vi "Error Converter (ErrCode or Status).vi"(8 "error in (no error)":errorcluster, 11 "error code":i32) -> (0 "error out":errorcluster)   [LabVIEW 2017, in "opcua.lvlib"]
uses:
  opcua.lvlib
panel:
  in  "string":string="This error is returned by the shared library function."
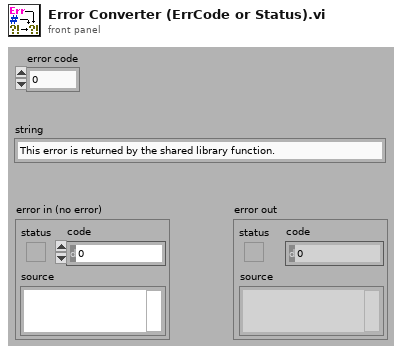
[diagram p1: front panel]
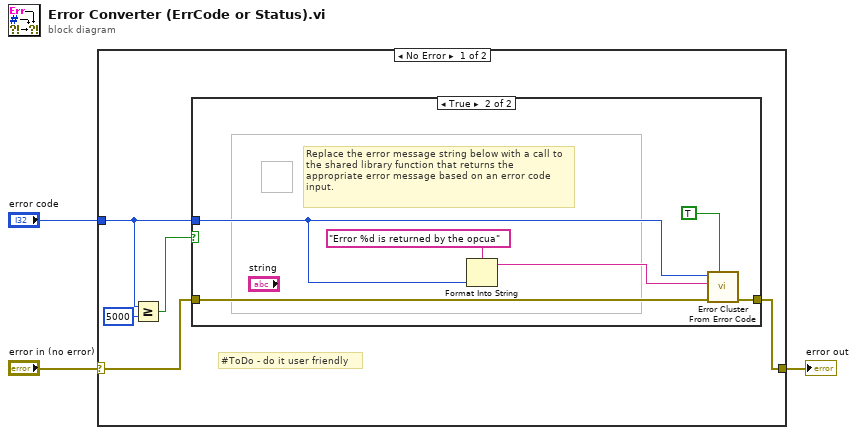
[diagram p0: block diagram]
diagram:
  n1 = case shown="No Error" "error in (no error)" {
    selector: "error in (no error)" -> [w8 w16]
    tunnel: [w7 w16] -> w2
    tunnel: "error code" -> [w6 _]
    frame No Error {
      # "#ToDo - do it user friendly"
      n2 = Greater Or Equal?(x=w6, y=5000) -> (x >= y?=w4:bool)
      n3 = case shown="True" w4 {
        tunnel: w8 -> [w9 w15]
        tunnel: w6 -> [_ w10]
        tunnel: [w9 w14] -> w7
        frame False {
        }
        frame True {
          # "Replace the error message string below with a call to the shared library function that returns the appropriate error message based on an error code input."
          n4 = Format Into String(format string="Error %d is returned by the opcua" ("string"), w10) -> (resulting string=w11:string)  [unwired: 2 in, 1 out]
          n5 = call <vilib>:"Error Cluster From Error Code.vi"("show call chain? (False)"=TRUE, "error in (no error)"=w15, "error message (\"\")"=w11, "error code (0)"=w10) -> ("error out"=w14:errorcluster)  [unwired: 5 in]
        }
      }
    }
    frame Error {
    }
  }
  "error out" <- w2
